vi "Master Data Handler 256-bit.vi"(0 "transfer settings":T2 {"Direction Change Bit" max=64 step=1; "Transfer Length (bits)" min=1 max=64 step=1}, 9 "controller interface":T1) -> (4 "shift MOSI":bool, 6 "sample MISO":bool, 8 "dir change":bool, 10 "read pending":bool, 15 "done":bool)   [LabVIEW 2015, in "SPI API.lvlib"]
doc: "This VI creates control signals to shift in MISO data and shift out MOSI data as well as determining when a transaction has completed."
uses:
  SPI API.lvlib
  Controls/Custom SPI IP U16 Transfer Settings.ctl
  Controls/Controller Interface.ctl
panel:
  # "This VI creates control signals to shift in MISO data and shift out MOSI data as well as determining when a transaction has completed."
  # "Controller interface cluster is simply a group of controls from the main SPI state machine. These controls are clustered for ease of use."
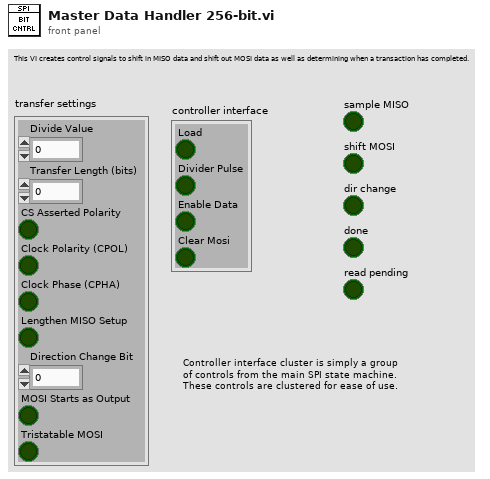
[diagram p1: front panel]
types:
  T1 = typedef "SPI API.lvlib/Controller Interface.ctl" = cluster{"Load":bool, "Divider Pulse":bool, "Enable Data":bool, "Clear Mosi":bool}
  T2 = typedef "SPI API.lvlib/Custom SPI IP U16 Transfer Settings.ctl" = cluster{"Divide Value":u8, "Transfer Length (bits)":u16, "CS Asserted Polarity":bool, "Clock Polarity (CPOL)":bool, "Clock Phase (CPHA)":bool, "Lengthen MISO Setup":bool, "Direction Change Bit":u8, "MOSI Starts as Output":bool, "Tristatable MOSI":bool}
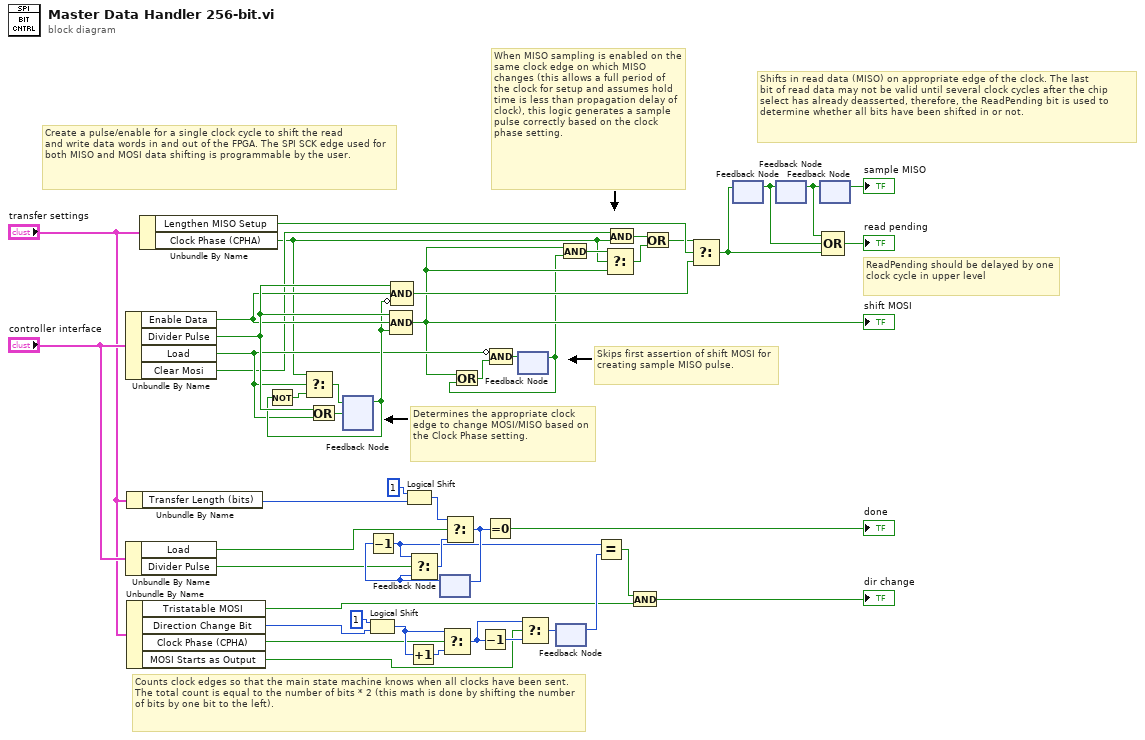
[diagram p0: block diagram]
diagram:
  # "Skips first assertion of shift MOSI for creating sample MISO pulse."
  # "When MISO sampling is enabled on the same clock edge on which MISO changes (this allows a full period of the clock for setup and assumes hold time is less than propagation delay of clock), this logic generates a sample pulse correctly based on the clock phase setting."
  # "Determines the appropriate clock edge to change MOSI/MISO based on the Clock Phase setting."
  # "Counts clock edges so that the main state machine knows when all clocks have been sent. The total count is equal to the number of bits * 2 (this math is done by shifting the number of bits by one bit to the left)."
  # "Create a pulse/enable for a single clock cycle to shift the read\nand write data words in and out of the FPGA. The SPI SCK edge used for both MISO and MOSI data shifting is programmable by the user."
  # "Shifts in read data (MISO) on appropriate edge of the clock. The last\nbit of read data may not be valid until several clock cycles after the chip select has already deasserted, therefore, the ReadPending bit is used to determine whether all bits have been shifted in or not."
  # "ReadPending should be delayed by one clock cycle in upper level"
  n1 = Unbundle By Name("controller interface") -> ("Enable Data"=w32:bool, "Divider Pulse"=w33:bool, "Load"=w24:bool, "Clear Mosi"=w23:bool)
  n2 = Unbundle By Name("controller interface") -> ("Load"=w43:bool, "Divider Pulse"=w44:bool)
  n3 = Unbundle By Name("transfer settings") -> ("Transfer Length (bits)"=w2:u16)
  n4 = Unbundle By Name("transfer settings") -> ("Tristatable MOSI"=w6:bool, "Direction Change Bit"=w1:u8, "Clock Phase (CPHA)"=w13:bool, "MOSI Starts as Output"=w8:bool)
  n5 = Unbundle By Name("transfer settings") -> ("Lengthen MISO Setup"=w30:bool, "Clock Phase (CPHA)"=w22:bool)
  n6 = Or(x=w33, y=w24) -> (x .or. y?=w36:bool)
  n7 = feedback #1() -> (w31:bool)  [unwired: 1 in]
  n8 = Not(x=w31) -> (.not. x?=w34:bool)
  n9 = Select(t=w22, s=w24, f=w34) -> (s? t:f=w35:bool)
  n10 = feedback-in #1(w35, w36) -> ()
  n11 = Logical Shift(y=i8 1, x=w1) -> (x << y=w16:u8)
  n12 = Compound Arithmetic op=AND(w33, w32, w31) -> (w4:bool)
  "shift MOSI" <- w4
  n13 = Compound Arithmetic op=AND(w33, w32, invert w31) -> (w29:bool)
  n14 = Logical Shift(y=i8 1, x=w2) -> (x << y=w47:u16)
  n15 = Increment(x=w16) -> (x+1=w15:u8)
  n16 = feedback #2() -> (w48:u16)  [unwired: 1 in]
  n17 = Decrement(x=w48) -> (x-1=w18:u16)
  n18 = Select(t=w18, s=w44, f=w48) -> (s? t:f=w46:u16)
  n19 = Select(t=w16, s=w13, f=w15) -> (s? t:f=w10:u8)
  n20 = Select(t=w47, s=w43, f=w46) -> (s? t:f=w19:u16)
  n21 = feedback-in #2(w19) -> ()
  n22 = Decrement(x=w10) -> (x-1=w11:u8)
  n23 = Equal To 0?(x=w19) -> (x = 0?=→"done":bool)
  n24 = feedback #3() -> (w3:bool)  [unwired: 1 in]
  n25 = Or(x=w4, y=w3) -> (x .or. y?=w39:bool)
  n26 = Compound Arithmetic op=AND(invert w24, w39) -> (w38:bool)
  n27 = feedback-in #3(w38) -> ()
  n28 = Select(t=w10, s=w8, f=w11) -> (s? t:f=w9:u8)
  n29 = feedback #4() -> (w14:u8)  [unwired: 1 in]
  n30 = feedback-in #4(w9) -> ()
  n31 = And(x=w4, y=w3) -> (x .and. y?=w26:bool)
  n32 = Equal?(x=w18, y=w14) -> (x = y?=w7:bool)
  n33 = Select(t=w26, s=w22, f=w4) -> (s? t:f=w25:bool)
  n34 = And(x=w23, y=w22) -> (x .and. y?=w21:bool)
  n35 = And(x=w7, y=w6) -> (x .and. y?=→"dir change":bool)
  n36 = Or(x=w21, y=w25) -> (x .or. y?=w27:bool)
  n37 = Select(t=w27, s=w30, f=w29) -> (s? t:f=w28:bool)
  n38 = feedback #5() -> (w40:bool)  [unwired: 1 in]
  n39 = feedback-in #5(w28) -> ()
  n40 = feedback #6() -> (w41:bool)  [unwired: 1 in]
  n41 = feedback-in #6(w40) -> ()
  n42 = feedback #7() -> (→"sample MISO":bool)  [unwired: 1 in]
  n43 = feedback-in #7(w41) -> ()
  n44 = Compound Arithmetic op=OR(w41, w40, w28) -> (→"read pending":bool)
